vi "Save Configuration.vi"(8 "error in (no error)":errorcluster, 11 "Configuration in":refnum<class "Configuration.lvclass">) -> (0 "error out":errorcluster, 3 "Configuration out":refnum<class "Configuration.lvclass">)   [LabVIEW 2023, in "Configuration.lvlib" / "Configuration.lvclass"]
uses:
  Library/Configuration.lvclass
  Library/Configuration.lvclass/Configuration.ctl
  <vilib>/Utility/config.llb/NI_LVConfig.lvlib
  <vilib>/Utility/config.llb/Write Key (String).vi
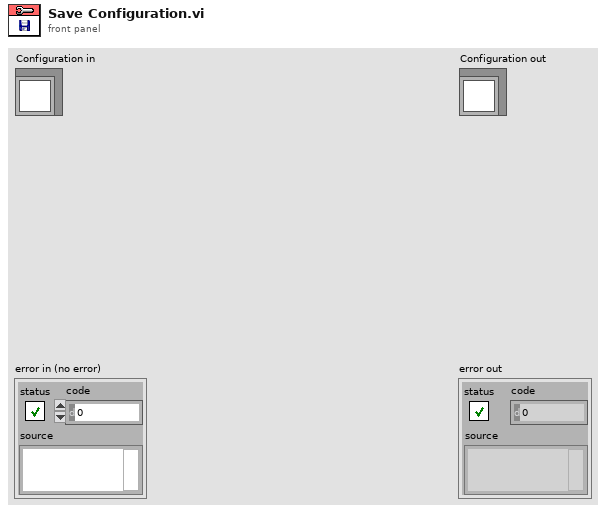
[diagram p1: front panel]
types:
  T1 = typedef "Configuration.lvlib/Configuration.lvclass/Definitions.ctl" = map{string, T2}
  T2 = typedef "Configuration.lvlib/Configuration.lvclass/Config.ctl" = map{string, string}
  T3 = typedef "NI_LVConfig.lvlib/Config Data RefNum.ctl" = refnum<k1>
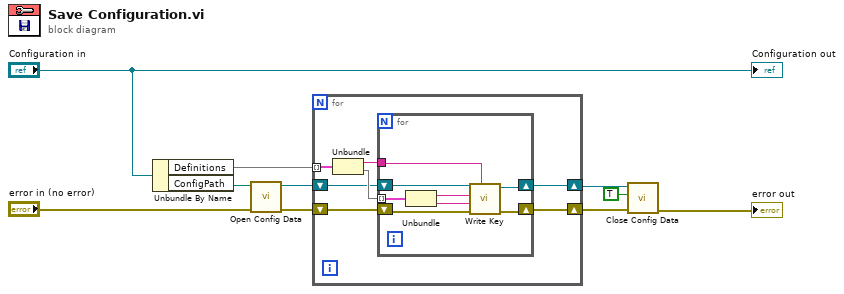
[diagram p0: block diagram]
diagram:
  n1 = Unbundle By Name("Configuration in") -> ("Definitions"=w10:T1, "ConfigPath"=w9:path)
  n2 = call <vilib>:"Open Config Data.vi"("error in (no error)"="error in (no error)", "configuration file path"=w9) -> ("error out"=w5:errorcluster, "refnum"=w8:T3)  [unwired: 7 in, 1 out]
  n3 = for {
    tunnel: w10 -> [w17] mode=indexing
    shift-right: [w13] -> w7
    shift-left: w8 -> [w14]
    shift-right: [w11] -> w3
    shift-left: w5 -> [w12]
    n4 = Unbundle(w17) -> ("Device"=w15:string, "Config"=w16:T2)
    n5 = for {
      tunnel: w16 -> [w25] mode=indexing
      tunnel: w15 -> [w20]
      shift-right: [w23] -> w13
      shift-left: w14 -> [w22]
      shift-right: [w24] -> w11
      shift-left: w12 -> [w21]
      n6 = Unbundle(w25) -> ("Key"=w19:string, "Value"=w18:string)
      n7 = call-poly <vilib>:"Write Key.vi"("section"=w20, "error in (no error)"=w21, "value"=w18, "key"=w19, "refnum"=w22) -> ("error out"=w24:errorcluster, "refnum out"=w23:T3)  [unwired: 4 in, 1 out]
    }
  }
  n8 = call <vilib>:"Close Config Data.vi"("error in (no error)"=w3, "write file if changed (T)"=TRUE, "refnum"=w7) -> ("error out"=→"error out":errorcluster)  [unwired: 7 in, 1 out]
  "Configuration out" <- "Configuration in"
